vi "find_consecutive_close_values.vi"(7 "module path":path=path "C:/Users/Taboada.r248/Documents/LabVIEW Projects/LabVIEW-2024-and-Python/pyhthon_modules/find_consecutive_close_values.py", 8 "error in (no error)":errorcluster, 9 "tolerance":dbl=4.0 format="%#_13g", 10 "min_threshold":dbl=5.0 format="%#_13g", 11 "data":dbl[](array[numeric])) -> (0 "error out":errorcluster, 1 "#_elements_found":i32, 2 "data qty":i32, 3 "Measures":dbl[][](array[numeric]), 4 "close_values":dbl[](array[numeric]) format="%.2f", 5 "average":dbl)   [LabVIEW 2024]
panel:
  # "Powered by \nPython 3.9.13\n32-bits"
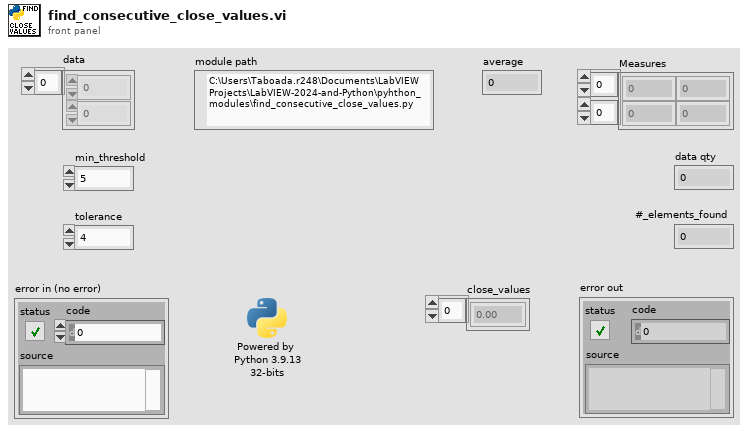
[diagram p1: front panel]
types:
  T1 = cluster{"close_values_w_zeros":dbl[], "num_elements_found":i32, "close_values":dbl[], "average":dbl}
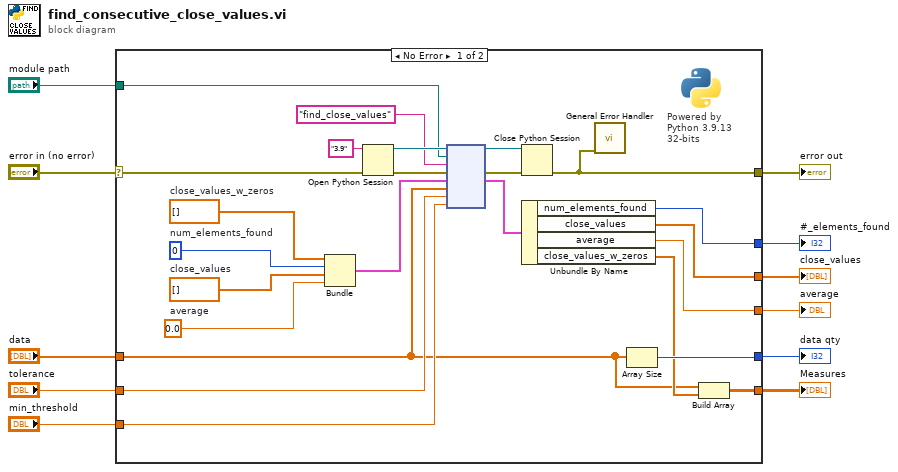
[diagram p0: block diagram]
diagram:
  n1 = case shown="No Error" "error in (no error)" {
    selector: "error in (no error)" -> [w17 w36]
    tunnel: "module path" -> [w30 _]
    tunnel: "min_threshold" -> [w23 _]
    tunnel: [w16 _] -> w9
    tunnel: [w15 _] -> w8
    tunnel: [w14 _] -> w7
    tunnel: [w21 _] -> w6
    tunnel: [w20 _] -> w1
    tunnel: "data" -> [w12 _]
    tunnel: "tolerance" -> [w19 _]
    tunnel: [w18 w36] -> w3
    frame No Error {
      w25 = 0.0  # average
      w26 = dbl[] []  # close_values
      w27 = 0  # num_elements_found
      w28 = dbl[] []  # close_values_w_zeros
      # "Powered by \nPython 3.9.13\n32-bits"
      n2 = Bundle("close_values_w_zeros"=w28, "num_elements_found"=w27, "close_values"=w26, "average"=w25) -> (w24:T1)  [unwired: 1 in]
      n3 = Open Python Session(python version="3.9" ("Python version"), 3:w17) -> (session out=w32:refnum<k35>, error out=w35:errorcluster)  [unwired: 1 in]
      n4 = node(w32, w30, "find_close_values" ("function name"), w35, w24, w12, w19, w23) -> (w31:refnum<k35>, w34:errorcluster, w22:T1)  [unwired: 3 in, 2 out]
      n5 = Close Python Session(session in=w31, error in=w34) -> (11:w18:errorcluster)
      n6 = Unbundle By Name(w22) -> ("num_elements_found"=w16:i32, "close_values"=w15:dbl[], "average"=w14:dbl, "close_values_w_zeros"=w13:dbl[])
      n7 = call <vilib>:"General Error Handler.vi"("error in (no error)"=w18) -> ()  [unwired: 10 in, 5 out]
      n8 = Array Size(array=w12) -> (size(s)=w21:i32)
      n9 = Build Array(w12, w13) -> (w20:dbl[][])
    }
    frame Error {
    }
  }
  "#_elements_found" <- w9
  "close_values" <- w8
  "average" <- w7
  "data qty" <- w6
  "Measures" <- w1
  "error out" <- w3
